vi "Pre Launch Init.vi"(11 "Actor_Log in":refnum<class "Actor_Log.lvclass">) -> (0 "error out":errorcluster, 3 "Actor_Log out":refnum<class "Actor_Log.lvclass">)   [LabVIEW 2020, in "Library Core.lvlib" / "Actor_Log.lvlib" / "Actor_Log.lvclass"]
doc: "(<B>Filename</B>: Actor Framework.lvlib:Actor.lvclass:Pre Launch Init.vi)\n\nDefines behavior that occurs after the Launch Nested Actor method is invoked but before the actor's Actor Core method begins running.\n\nBy default, this method does nothing. A descendant class may override it to define behavior."
uses:
  Actor_Log.lvclass
  C:/Program Files (x86)/National Instruments/LabVIEW 2020/vi.lib/ActorFramework/Actor/Actor.lvclass
  Actor_Log.lvclass/Actor_Log.ctl
  <vilib>/ActorFramework/Actor/Actor.lvclass/Actor.ctl
  <vilib>/ActorFramework/Message Enqueuer/Message Enqueuer.lvclass/Message Enqueuer.ctl
  <vilib>/ActorFramework/Message Enqueuer/Init from Existing Queue.vi
  <vilib>/ActorFramework/Message Enqueuer/Enqueue.vi
  <vilib>/ActorFramework/Stop Msg/Stop Msg.lvclass
  C:/Program Files (x86)/National Instruments/LabVIEW 2020/vi.lib/ActorFramework/Message/Message.lvclass
  <vilib>/ActorFramework/Message Priority Queue/Priority Enqueue.vi
  <vilib>/ActorFramework/Message Enqueuer/Message Enqueuer.lvclass
  <vilib>/ActorFramework/Actor/Actor.lvclass
  Commun VI/Library Commun.lvlib
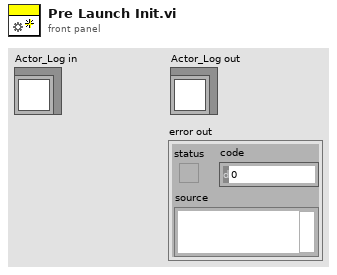
[diagram p1: front panel]
types:
  T1 = enum16{"Init", "Add Actor", "Delete Actor", "Get Actor Queue", "Get Log Actor Queue", "List all actors"}
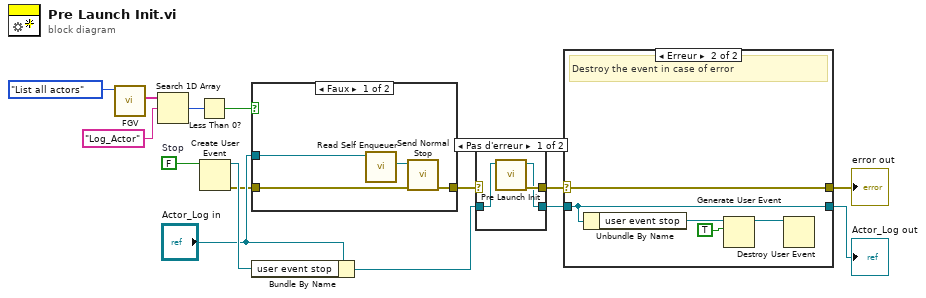
[diagram p0: block diagram]
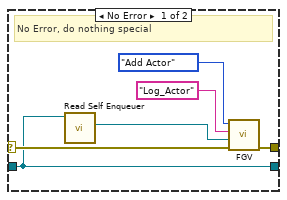
[diagram p3: hidden frame]
diagram:
  w15 = FALSE  # Stop
  n1 = call "FGV.vi"("Action"=T1."List all actors") -> ("Actor names"=w8:string[])  [unwired: 8 in, 2 out]
  n2 = Search 1D Array(1D array=w8, element="Log_Actor") -> (index of element=w6:i32)  [unwired: 1 in]
  n3 = Less Than 0?(x=w6) -> (x < 0?=w1:bool)
  n4 = Create User Event(user event datatype=w15) -> (user event=w5:refnum<user-event>, error out=w3:errorcluster)  [unwired: 1 in]
  n5 = case shown="Faux" w1 {
    tunnel: "Actor_Log in" -> [w19 _]
    tunnel: w3 -> [w17 w20]
    tunnel: [w16 w20] -> w2
    frame False {
      n6 = call <vilib>:"Read Self Enqueuer.vi"("Actor"=w19) -> ("Self Enqueuer"=w18:refnum<class "Message Enqueuer.lvclass">)  [unwired: 10 in]
      n7 = call <vilib>:"Send Normal Stop.vi"("error in (no error)"=w17, "Message Enqueuer"=w18) -> ("error out"=w16:errorcluster)  [unwired: 9 in]
    }
    frame True {
    }
  }
  n8 = Bundle By Name(cluster="Actor_Log in", "user event stop"=w5) -> (w14:refnum<class "Actor_Log.lvclass">)
  n9 = case shown="Pas d'erreur" w2 {
    selector: w2 -> [_ w25]
    tunnel: [w23 w25] -> w13
    tunnel: w14 -> [w22 w24]
    tunnel: [w21 w24] -> w12
    frame No Error {
      n10 = call-parent "Pre Launch Init.vi"("Actor in"=w22) -> ("error out"=w23:errorcluster, "Actor out"=w21:refnum<class "Actor_Log.lvclass">)  [unwired: 9 in]
    }
    frame Error {
    }
  }
  n11 = case shown="Erreur" w13 {
    selector: w13 -> [w30 w32]
    tunnel: w12 -> [w28 w33]
    tunnel: [w29 w32] -> w11
    tunnel: [w28 w33] -> w10
    frame No Error {
      # "No Error, do nothing special"
      n12 = call <vilib>:"Read Self Enqueuer.vi"("Actor"=w28) -> ("Self Enqueuer"=w27:refnum<class "Message Enqueuer.lvclass">)  [unwired: 10 in]
      n13 = call "FGV.vi"("error in (no error)"=w30, "Actor's Queue In"=w27, "Actor name"="Log_Actor", "Action"=T1."Add Actor") -> ("error out"=w29:errorcluster)  [unwired: 5 in, 2 out]
    }
    frame Error {
      # "Destroy the event in case of error"
      n14 = Unbundle By Name(w33) -> ("user event stop"=w36:refnum<user-event>)
      n15 = Generate User Event(user event=w36, event data cluster=TRUE ("event data")) -> (user event out=w34:refnum<user-event>)  [unwired: 2 in, 1 out]
      n16 = Destroy User Event(user event=w34) -> ()  [unwired: 1 in, 1 out]
    }
  }
  "error out" <- w11
  "Actor_Log out" <- w10
